vi "temperature_watcher.vi"(1 "Port Number":u16=32541, 2 "Command":T1(ring)=enum."sorb_temp") -> (0 "Response":string)   [LabVIEW 2010]
panel:
  # "Temperature Watcher"
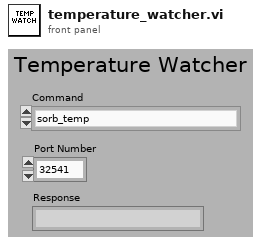
[diagram p1: front panel]
types:
  T1 = enum16{"pot_temp", "sorb_temp", "needle_valve_temp", "still_temp", "mix_chamber_temp", "stm_rx_temp", "stm_cx_temp", "tank_pressure", "condense_pressure", "still_pressure", "turbo_back_pressure", "n2_trap_pressure"}
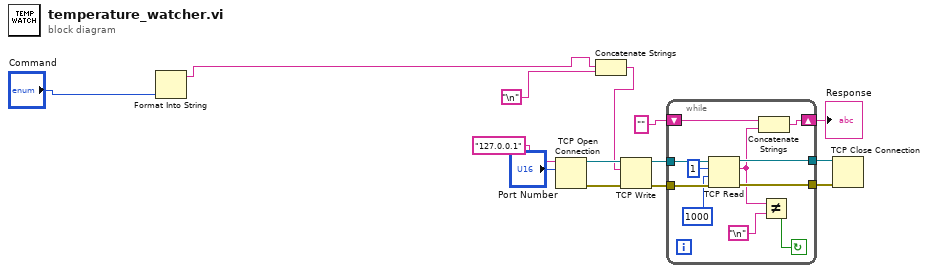
[diagram p0: block diagram]
diagram:
  n1 = Format Into String("Command") -> (resulting string=w3:string)  [unwired: 3 in, 1 out]
  n2 = TCP Open Connection(address="127.0.0.1", remote port or service name="Port Number") -> (connection ID=w13:refnum<k5>, error out=w12:errorcluster)  [unwired: 3 in]
  n3 = Concatenate Strings(w3, "\n") -> (w5:string)
  n4 = TCP Write(connection ID=w13, data in=w5, error in (no error)=w12) -> (connection ID out=w10:refnum<k5>, error out=w11:errorcluster)  [unwired: 1 in, 1 out]
  n5 = while {
    tunnel: w11 -> [w25]
    tunnel: w10 -> [w24]
    tunnel: [w23] -> w9
    tunnel: [w22] -> w8
    shift-right: [w18] -> w6
    shift-left: "" ("string") -> [w19]
    stop <- w17 continue-if-true
    n6 = TCP Read(connection ID=w24, bytes to read=1, error in (no error)=w25, 9:1000 ("timeout ms (25000)")) -> (connection ID out=w22:refnum<k5>, data out=w16:string, error out=w23:errorcluster)  [unwired: 1 in]
    n7 = Concatenate Strings(w19, w16) -> (w18:string)
    n8 = Not Equal?(x=w16, y="\n") -> (x != y?=w17:bool)
  }
  "Response" <- w6
  n9 = TCP Close Connection(connection ID=w8, error in (no error)=w9) -> ()  [unwired: 1 in, 2 out]
